vi "merge single fault.vi"(10 "new fault":T1, 11 "all faults in":T3[](array[typedef])) -> (3 "all faults out":T3[](array[typedef]))   [LabVIEW 2013, in "main engine.lvlib"]
uses:
  main engine/main engine.lvlib
  <vilib>/NI/Module Execution Interface/Engine Runtime/Fault.ctl
  <vilib>/NI/Tag Bus Module Framework/runtime/error classification.ctl
  rt fault.ctl
  <vilib>/NI/Tag Bus Module Framework/module configuration/TBM module configuration.lvclass
  <vilib>/NI/Configuration Framework/serializable configuration/NISE_CEF_serializable configuration.lvclass/NISE_CEF_serializable configuration.ctl
  <vilib>/NI/Configuration Framework/serializable configuration/NISE_CEF_serializable configuration.lvclass
  <vilib>/NI/Tag Bus Module Framework/runtime/TBM module execution interface.lvclass
  <vilib>/NI/Module Execution Interface/Engine Runtime/Engine Runtime Interface.lvclass
  worker pool.lvlib
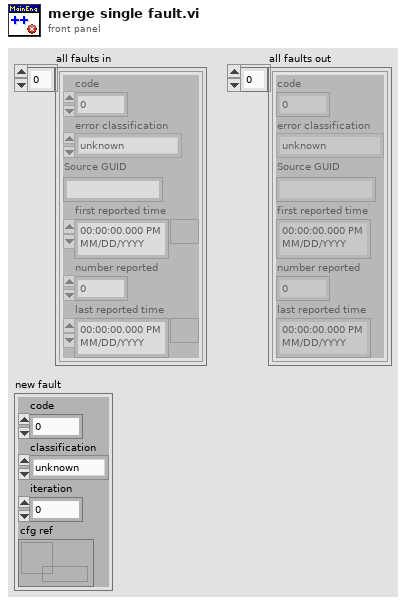
[diagram p1: front panel]
types:
  T1 = typedef "worker pool.lvlib/rt fault.ctl" = cluster{"code":i32, "classification":T2, "iteration":u64, "cfg ref":refnum<data-value>}
  T2 = typedef "TBM module execution interface.lvclass/error classification.ctl" = enum16{"unknown", "none", "trivial", "recoverable", "critical"}
  T3 = typedef "Engine Runtime Interface.lvclass/Fault.ctl" = cluster{"code":i32, "error classification":T2, "Source GUID":string, "first reported time":timestamp, "number reported":u32, "last reported time":timestamp}
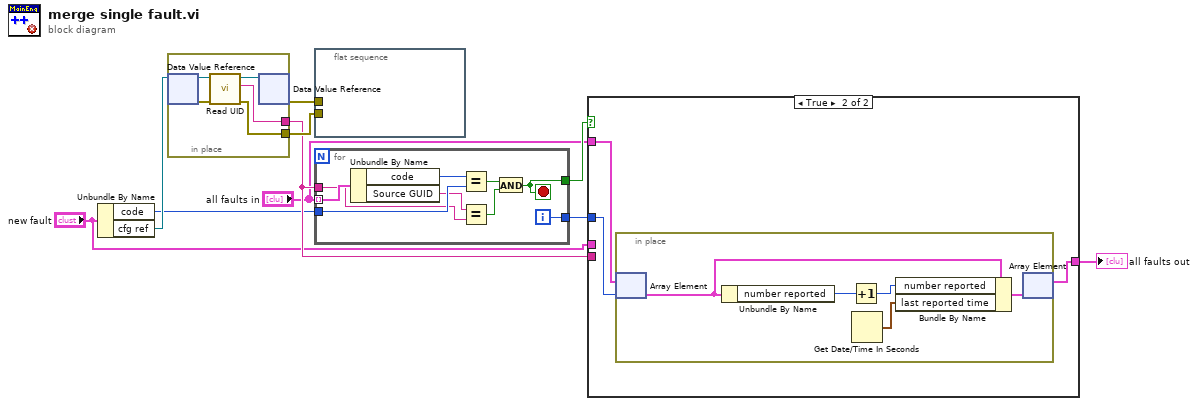
[diagram p0: block diagram]
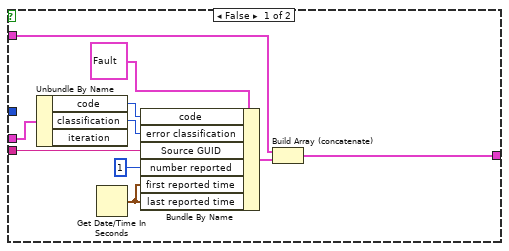
[diagram p2: hidden frame]
diagram:
  n1 = Unbundle By Name("new fault") -> ("code"=w1:i32, "cfg ref"=w5:refnum<data-value>)
  n2 = in-place {
    in-place-border: [w12] -> w6
    in-place-border: [w11] -> w10
    n3 = in-place-dvr #1(w5) -> (w15:refnum<class "TBM module configuration.lvclass">, w13:errorcluster)
    n4 = call <vilib>:"Read UID.vi"("error in"=w13, "configuration in"=w15) -> ("error out"=w11:errorcluster, "instance id"=w12:string, "configuration out"=w14:refnum<class "TBM module configuration.lvclass">)  [unwired: 7 in]
    n5 = in-place-dvr #1(w14) -> (w9:errorcluster)  [unwired: 1 out]
  }
  n6 = flat-sequence {
    tunnel: w9 -> [_]
    tunnel: w10 -> [_]
    frame #0 {
    }
  }
  n7 = for {
    tunnel: "all faults in" -> [w24] mode=indexing
    tunnel: w1 -> [w22]
    tunnel: w6 -> [w21]
    tunnel: [w17] -> w8
    tunnel: [w16] -> w7
    i -> [w17]
    stop <- w16 stop-if-true
    n8 = Unbundle By Name(w24) -> ("code"=w23:i32, "Source GUID"=w20:string)
    n9 = Equal?(x=w23, y=w22) -> (x = y?=w19:bool)
    n10 = Equal?(x=w20, y=w21) -> (x = y?=w18:bool)
    n11 = And(x=w19, y=w18) -> (x .and. y?=w16:bool)
  }
  n12 = case shown="True" w7 {
    tunnel: "new fault" -> [w30 _]
    tunnel: w6 -> [w27 _]
    tunnel: w8 -> [_ w36]
    tunnel: "all faults in" -> [w34 w37]
    tunnel: [w33 w35] -> w4
    frame False {
      n13 = Unbundle By Name(w30) -> ("code"=w28:i32, "classification"=w29:T2)  [unwired: 1 out]
      n14 = Get Date/Time In Seconds() -> (seconds since 1Jan1904=w25:timestamp)
      n15 = Bundle By Name(cluster=T3 {"code"=0, "error classification"=enum."unknown", "Source GUID"="", "first reported time"=timestamp(0 s since 1904-01-01), "number reported"=0, "last reported time"=timestamp(0 s since 1904-01-01)} ("fault"), "code"=w28, "error classification"=w29, "Source GUID"=w27, "number reported"=u32 1, "first reported time"=w25, "last reported time"=w25) -> (w31:T3)
      n16 = Build Array (concatenate)(w34, w31) -> (w33:T3[])
    }
    frame True {
      n17 = in-place {
        n18 = in-place-array #2(w37, w36) -> (w42:T3)
        n19 = Unbundle By Name(w42) -> ("number reported"=w40:u32)
        n20 = Increment(x=w40) -> (x+1=w38:u32)
        n21 = Get Date/Time In Seconds() -> (seconds since 1Jan1904=w39:timestamp)
        n22 = Bundle By Name(cluster=w42, "number reported"=w38, "last reported time"=w39) -> (w41:T3)
        n23 = in-place-array #2(w41) -> (w35:T3[])  [unwired: 1 out]
      }
    }
  }
  "all faults out" <- w4
